vi "GlobalBooleans.vi"(2 "Write Value":bool, 3 "Element":i32, 4 "Operation":i32 min=0 max=1, 5 "Number of Elements":i32=30) -> (0 "Boolean Array Out":bool[](array[boolean]), 1 "Read Value":bool)   [LabVIEW 2015]
doc: "Handle Boolean Globals Style II.\nThe globals are maintained in a \nshift register, as an array of booleans.\nTherefore, It is mandatory to initialize the\narray with a first invocation wiring the\nnumber of elements to be contained\nin the array. The elements witl be\ninitialized to FALSE\n\n\nINPUTS:\n Number of Elements: Use only on first call to\n initialize the array.\n Operation: 1 = WRITE, 0 = READ\n Element: Element of the array to write or read\n Write Value: Boolean value to store\nOUTPUTS:\n Read Value: Boolean value retrieved\n Boolean Array Out: The entire array of booleans"
panel:
  # "1 =  WRITE"
  # "0 = READ"
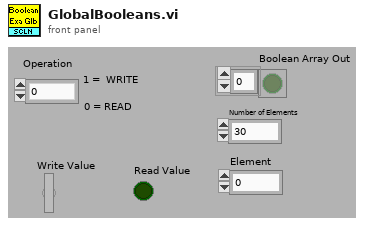
[diagram p1: front panel]
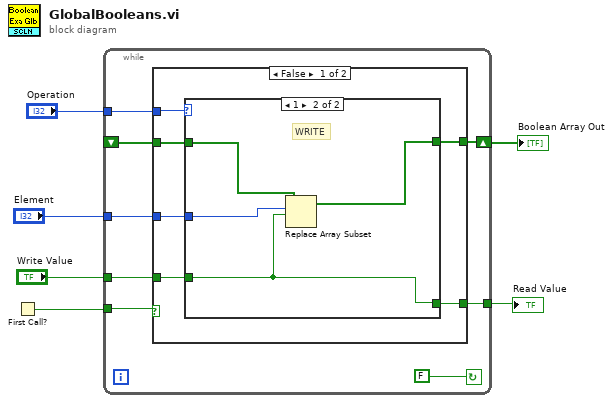
[diagram p0: block diagram]
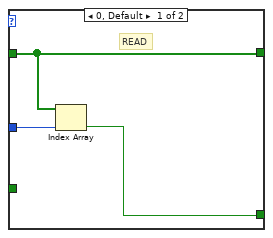
[diagram p2: hidden frame]
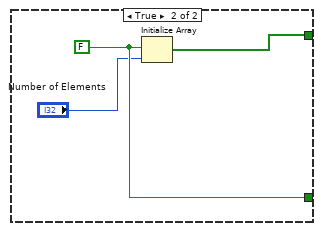
[diagram p3: hidden frame]
diagram:
  n1 = First Call?() -> (First Call?: T/F=w1:bool)
  n2 = while {
    tunnel: "Operation" -> [w13]
    shift-right: [w12] -> w2
    shift-left: _ -> [w11]
    tunnel: "Element" -> [w10]
    tunnel: "Write Value" -> [w9]
    tunnel: [w8] -> w3
    tunnel: w1 -> [w7]
    stop <- FALSE continue-if-true
    n3 = case shown="False" w7 {
      tunnel: w13 -> [w20 _]
      tunnel: [w19 w30] -> w12
      tunnel: w11 -> [w18 _]
      tunnel: w10 -> [w17 _]
      tunnel: w9 -> [w16 _]
      tunnel: [w15 w29] -> w8
      frame False {
        n4 = case shown="1" w20 {
          tunnel: [w21 w25] -> w19
          tunnel: w18 -> [w21 w24]
          tunnel: w17 -> [w23 w26]
          tunnel: w16 -> [_ w27]
          tunnel: [w22 w27] -> w15
          frame 0, Default {
            # "READ"
            n5 = Index Array(array=w21, index=w23) -> (element=w22:bool)
          }
          frame 1 {
            # "WRITE"
            n6 = Replace Array Subset(array=w24, new element=w27, index=w26) -> (w25:bool[])
          }
        }
      }
      frame True {
        w29 = FALSE
        n7 = Initialize Array(w29, "Number of Elements") -> (w30:bool[])
      }
    }
  }
  "Read Value" <- w3
  "Boolean Array Out" <- w2
